vi "Create NI-DCPower Session.vi"(8 "error in (no error)":errorcluster, 10 "session information":T3, 11 "gRPC channel pool":T1) -> (0 "error out":errorcluster, 2 "instrument handle":refnum<k15>, 3 "gRPC channel pool out":T1)   [LabVIEW 2020, in "NIDCPowerSourceDCVoltage.lvlib"]
doc: "Creates and returns an gRPC based NI DC power instrument handle."
uses:
  NIDCPowerSourceDCVoltage.lvlib
  <vilib>/MeasurementLink/MeasurementLink Session Management Client/RPC Messages/ni_measurementlink_sessionmanagement_v1_SessionInformation.ctl
  <vilib>/MeasurementLink/MeasurementLink Session Management Client/RPC Messages/nidevice_grpc_Session.ctl
  <vilib>/MeasurementLink/MeasurementLink Session Management Client/RPC Messages/ni_measurementlink_sessionmanagement_v1_ChannelMapping.ctl
  GRPC Clients.ctl
  <vilib>/gRPC/LabVIEW gRPC Library/Shared/grpcId.ctl
  <vilib>/MeasurementLink/MeasurementLink Session Management Client/MeasurementLink Session Management Client.lvlib
  <vilib>/gRPC/LabVIEW gRPC Library/grpc-lvsupport-release.lvlib
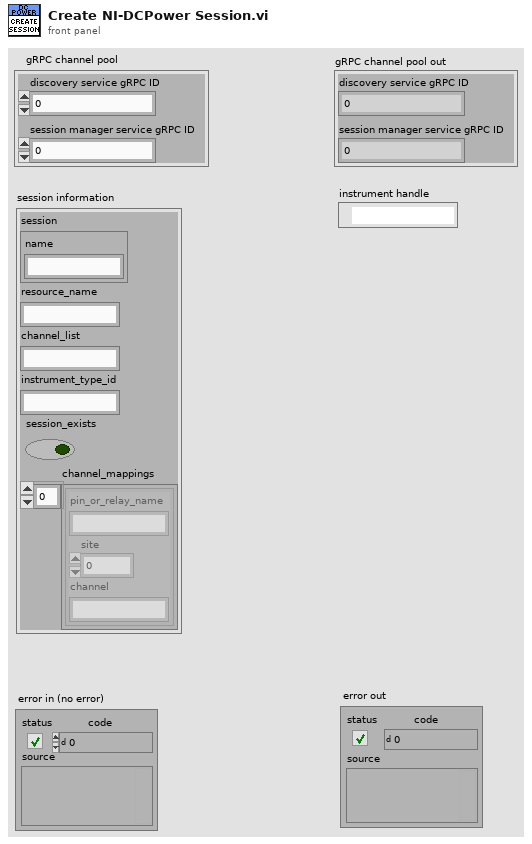
[diagram p1: front panel]
types:
  T1 = typedef "NIDCPowerSourceDCVoltage.lvlib/GRPC Clients.ctl" = cluster{"discovery service gRPC ID":T2, "session manager service gRPC ID":T2}
  T2 = typedef "grpc-lvsupport-release.lvlib/grpcId.ctl" = u64
  T3 = typedef "MeasurementLink Session Management Client.lvlib/ni_measurementlink_sessionmanagement_v1_SessionInformation.ctl" = cluster{"session":T4, "resource_name":string, "channel_list":string, "instrument_type_id":string, "session_exists":bool, "channel_mappings":T5[]}
  T4 = typedef "MeasurementLink Session Management Client.lvlib/nidevice_grpc_Session.ctl" = cluster{"name":string}
  T5 = typedef "MeasurementLink Session Management Client.lvlib/ni_measurementlink_sessionmanagement_v1_ChannelMapping.ctl" = cluster{"pin_or_relay_name":string, "site":i32, "channel":string}
  T6 = typedef "MeasurementLink Discovery Client.lvlib/ni_measurementlink_discovery_v1_ServiceLocation.ctl" = cluster{"location":string, "insecure_port":string, "ssl_authenticated_port":string}
  T7 = typedef "niDCPower gRPC Device Server.ctl" = cluster{"session name":string, "address (localhost)":string, "port (31763)":u32}
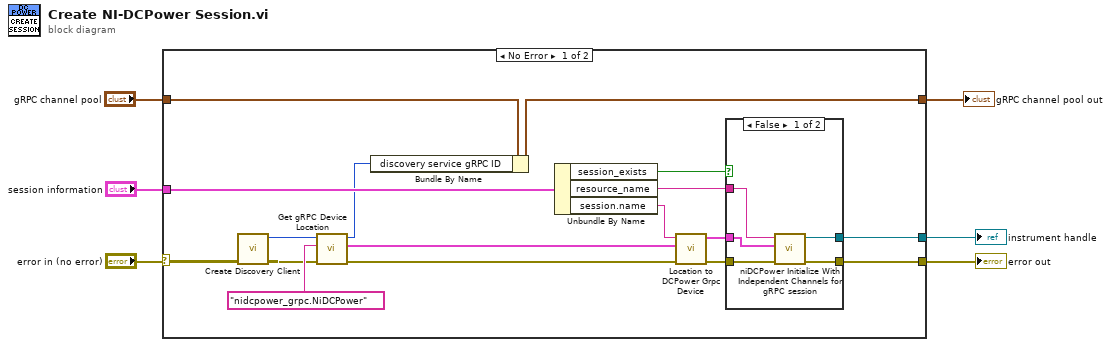
[diagram p0: block diagram]
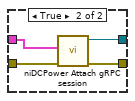
[diagram p2: hidden frame]
diagram:
  n1 = case shown="No Error" "error in (no error)" {
    selector: "error in (no error)" -> [w15 w33]
    tunnel: "session information" -> [w22 _]
    tunnel: [w17 w33] -> w5
    tunnel: [w16 _] -> w4
    tunnel: "gRPC channel pool" -> [w9 w32]
    tunnel: [w8 w32] -> w1
    frame No Error {
      n2 = call "Create Discovery Client.vi"("error in"=w15) -> ("error out"=w11:errorcluster, "discovery service gRPC ID Out"=w10:T2)  [unwired: 9 in]
      n3 = call "Get gRPC Device Location.vi"("error in"=w11, "provided_interface"="nidcpower_grpc.NiDCPower", "discovery service gRPC ID"=w10) -> ("error out"=w14:errorcluster, "gRPC device location"=w12:T6, "discovery service gRPC ID out"=w7:T2)  [unwired: 6 in]
      n4 = Bundle By Name(cluster=w9, "discovery service gRPC ID"=w7) -> (w8:T1)
      n5 = Unbundle By Name(w22) -> ("session_exists"=w21:bool, "resource_name"=w18:string, "session.name"=w20:string)
      n6 = call "Location to DCPower Grpc Device.vi"("Grpc Device Location"=w12, "Session Name"=w20) -> ("NI gRPC Device Server Out"=w19:T7)  [unwired: 9 in]
      n7 = case shown="False" w21 {
        tunnel: w19 -> [w25 w29]
        tunnel: w18 -> [w24 _]
        tunnel: w14 -> [w27 w31]
        tunnel: [w26 w30] -> w17
        tunnel: [w23 w28] -> w16
        frame False {
          n8 = call <instrlib>:"niDCPower Initialize With Independent Channels for gRPC session.vi"("error in (no error)"=w27, "gRPC options"=w25, "resource name"=w24) -> ("error out"=w26:errorcluster, "instrument handle out"=w23:refnum<k15>)  [unwired: 7 in]
        }
        frame True {
          n9 = call <instrlib>:"niDCPower Attach gRPC session.vi"("error in (no error)"=w31, "gRPC options"=w29) -> ("error out"=w30:errorcluster, "instrument handle out"=w28:refnum<k15>)  [unwired: 8 in]
        }
      }
    }
    frame Error {
    }
  }
  "instrument handle" <- w4
  "error out" <- w5
  "gRPC channel pool out" <- w1
